vi "log analysis_gps.vi"() -> ()   [LabVIEW 2019] (continued)
INS_RTKFIXED,37.37053109061,126.72444506207,11.0879,22.3000,0.1993,-0.2262,-0.0239,-0.578200163,-2.123585690,301.384652379,0.4420,0.2933,0.5470,0.1138,0.0924,0.0770,0.0993,0.1038,4.8409,0f000001,0*2eda5995\n\t", "INSPVAXA,USB3,0,45.5,FINESTEERING,2107,282664.900,02000000,471d,15824;INS_ALIGNMENT_COMPLETE,INS_RTKFIXED,37.37053183209,126.72444381821,11.0830,22.3000,0.2025,-0.2395,-0.0183,-0.627563942,-2.176125382,301.462972604,0.4420,0.2933,0.5470,0.1138,0.0924,0.0770,0.0993,0.1038,4.8409,0f000001,0*51325076\n\t", "INSPVAXA,USB3,0,50.5,FINESTEERING,2107,282665.400,02000000,471d,15824;INS_ALIGNMENT_COMPLETE,INS_RTKFIXED,37.37053260836,126.72444247630,11.0777,22.3000,0.1697,-0.2000,-0.0233,-0.806380731,-2.428315608,301.586666898,0.4420,0.2935,0.5472,0.1137,0.0923,0.0770,0.0992,0.1038,4.8415,0f000001,0*d8a31360\n\t", "INSPVAXA,USB3,0,50.5,FINESTEERING,2107,282665.900,02000000,471d,15824;INS_ALIGNMENT_COMPLETE,INS_RTKFIXED,37.37053337130,126.72444116871,11.0726,22.3000,0.1954,-0.2209,-0.0080,-0.903161753,-2.476998563,301.699215129,0.4420,0.2935,0.5472,0.1137,0.0923,0.0770,0.0992,0.1038,4.8415,0f000001,0*b607e80f\n\t", "DUALANTENNAHEADINGA,USB3,0,47.0,FINESTEERING,2107,282666.400,02000000,d426,15824;INSUFFICIENT_OBS,NONE,-1.000000000,0.000000000,0.000000000,0.0,0.000000000,0.000000000,\"631T\",14,3,3,3,04,00,20,00*a6710081\n\t", "INSPVAXA,USB3,0,47.0,FINESTEERING,2107,282666.900,02000000,471d,15824;INS_ALIGNMENT_COMPLETE,INS_RTKFIXED,37.37053484048,126.72443859916,11.0582,22.3000,0.1830,-0.2119,-0.0311,-0.968807751,-2.464707022,301.855553753,0.4415,0.2935,0.5473,0.1137,0.0925,0.0771,0.0992,0.1038,4.8423,0f000001,0*59f4e239\n\t", "DUALANTENNAHEADINGA,USB3,0,49.5,FINESTEERING,2107,282667.400,02000000,d426,15824;INSUFFICIENT_OBS,NONE,-1.000000000,0.000000000,0.000000000,0.0,0.000000000,0.000000000,\"631T\",15,3,3,3,04,00,20,00*5f1e2af7\n\t", "INSPVAXA,USB3,0,49.5,FINESTEERING,2107,282667.900,02000000,471d,15824;INS_ALIGNMENT_COMPLETE,INS_RTKFIXED,37.37053633502,126.72443604770,11.0435,22.3000,0.1822,-0.2080,-0.0221,-0.962443537,-2.273211285,302.003209651,0.4405,0.2936,0.5472,0.1136,0.0924,0.0770,0.0991,0.1038,4.8429,0f000001,0*2d8cca71\n\t", "DUALANTENNAHEADINGA,USB3,0,51.0,FINESTEERING,2107,282668.400,02000000,d426,15824;INSUFFICIENT_OBS,NONE,-1.000000000,0.000000000,0.000000000,0.0,0.000000000,0.000000000,\"631T\",13,3,3,3,04,00,20,00*d0f86fa9\n\t", "INSPVAXA,USB3,0,51.0,FINESTEERING,2107,282668.900,02000000,471d,15824;INS_ALIGNMENT_COMPLETE,INS_RTKFIXED,37.37053784422,126.72443343900,11.0314,22.3000,0.1770,-0.2175,-0.0238,-1.067658542,-2.117354473,302.168245726,0.4406,0.2938,0.5474,0.1136,0.0926,0.0771,0.0991,0.1038,4.8433,0f000001,0*743eb533\n\t", "INSPVAXA,USB3,0,50.5,FINESTEERING,2107,282669.400,02000000,471d,15824;INS_ALIGNMENT_COMPLETE,INS_RTKFIXED,37.37053859261,126.72443216227,11.0246,22.3000,0.1748,-0.2150,-0.0262,-1.134800808,-1.987218323,302.206484559,0.4410,0.2939,0.5476,0.1137,0.0929,0.0771,0.0990,0.1039,4.8430,0f000001,0*0ef77350\n\t", "INSPVAXA,USB3,0,50.5,FINESTEERING,2107,282669.900,02000000,471d,15824;INS_ALIGNMENT_COMPLETE,INS_RTKFIXED,37.37053936070,126.72443086861,11.0170,22.3000,0.1679,-0.2152,-0.0201,-1.047863329,-2.047137616,302.259088217,0.4410,0.2939,0.5476,0.1137,0.0929,0.0771,0.0990,0.1039,4.8430,0f000001,0*b3a345e1\n\t", "INSPVAXA,USB3,0,51.5,FINESTEERING,2107,282670.400,02000000,471d,15824;INS_ALIGNMENT_COMPLETE,INS_RTKFIXED,37.37054013304,126.72442955163,11.0107,22.3000,0.1797,-0.2154,-0.0330,-1.008775367,-2.075430336,302.292083469,0.4412,0.2940,0.5477,0.1137,0.0927,0.0771,0.0989,0.1039,4.8414,0f000001,0*6124701b\n\t", "INSPVAXA,USB3,0,51.5,FINESTEERING,2107,282670.900,02000000,471d,15824;INS_ALIGNMENT_COMPLETE,INS_RTKFIXED,37.37054088934,126.72442826376,11.0051,22.3000,0.1741,-0.2301,-0.0351,-1.043464274,-1.977986056,302.323016199,0.4412,0.2940,0.5477,0.1137,0.0927,0.0771,0.0989,0.1039,4.8414,0f000001,0*5cd64784\n\t", "INSPVAXA,USB3,0,51.0,FINESTEERING,2107,282671.400,02000000,471d,15824;INS_ALIGNMENT_COMPLETE,INS_RTKFIXED,37.37054164500,126.72442698236,10.9999,22.3000,0.1651,-0.2207,-0.0264,-1.152870335,-2.003288963,302.368323626,0.4421,0.2942,0.5481,0.1138,0.0926,0.0771,0.0989,0.1039,4.8395,0f000001,0*729e65cc\n\t", "DUALANTENNAHEADINGA,USB3,0,51.0,FINESTEERING,2107,282671.900,02000000,d426,15824;SOL_COMPUTED,L1_FLOAT,-1.000000000,6.424537182,-37.266357422,0.0,360.000000000,180.000000000,\"631T\",14,5,5,5,04,00,20,20*1315aa76\n\t", "INSPVAXA,USB3,0,52.5,FINESTEERING,2107,282672.400,02000000,471d,15824;INS_ALIGNMENT_COMPLETE,INS_RTKFIXED,37.37054317479,126.72442436870,10.9904,22.3000,0.1725,-0.2321,-0.0318,-1.253314249,-1.912910767,302.408086274,0.4431,0.2945,0.5488,0.1140,0.0927,0.0771,0.0988,0.1039,4.8375,0f000001,0*4ca87b98\n\t", "INSPVAXA,USB3,0,52.5,FINESTEERING,2107,282672.900,02000000,471d,15824;INS_ALIGNMENT_COMPLETE,INS_RTKFIXED,37.37054392116,126.72442309351,10.9862,22.3000,0.1660,-0.2327,-0.0240,-1.192361701,-1.928177514,302.476152160,0.4431,0.2945,0.5488,0.1140,0.0927,0.0771,0.0988,0.1039,4.8375,0f000001,0*83cc3094\n\t", "INSPVAXA,USB3,0,51.5,FINESTEERING,2107,282673.400,02000000,471d,15824;INS_ALIGNMENT_COMPLETE,INS_RTKFIXED,37.37054468191,126.72442179361,10.9818,22.3000,0.1549,-0.2194,-0.0237,-1.138544711,-1.857754611,302.526216112,0.4445,0.2949,0.5496,0.1141,0.0925,0.0772,0.0988,0.1040,4.8352,0f000001,0*601d5af9\n\t", "INSPVAXA,USB3,0,51.5,FINESTEERING,2107,282673.900,02000000,471d,15824;INS_ALIGNMENT_COMPLETE,INS_RTKFIXED,37.37054544133,126.72442048455,10.9776,22.3000,0.1608,-0.2204,-0.0208,-1.194325383,-1.773338448,302.575514269,0.4445,0.2949,0.5496,0.1141,0.0925,0.0772,0.0988,0.1040,4.8352,0f000001,0*3c4b28bd\n\t", "DUALANTENNAHEADINGA,USB3,0,52.0,FINESTEERING,2107,282674.400,02000000,d426,15824;INSUFFICIENT_OBS,NONE,-1.000000000,0.000000000,0.000000000,0.0,0.000000000,0.000000000,\"631T\",11,3,3,3,04,00,20,00*43d09faf\n\t", "INSPVAXA,USB3,0,52.0,FINESTEERING,2107,282674.900,02000000,471d,15824;INS_ALIGNMENT_COMPLETE,INS_RTKFIXED,37.37054694617,126.72441789266,10.9675,22.3000,0.1711,-0.2297,-0.0188,-1.275138168,-1.781517765,302.710392132,0.4449,0.2948,0.5501,0.1143,0.0927,0.0772,0.0987,0.1040,4.8338,0f000001,0*704fcea3\n\t", "INSPVAXA,USB3,0,50.5,FINESTEERING,2107,282675.400,02000000,471d,15824;INS_ALIGNMENT_COMPLETE,INS_RTKFIXED,37.37054775333,126.72441659154,10.9642,22.3000,0.1645,-0.2327,-0.0094,-1.051395479,-1.879417233,302.757545593,0.4453,0.2948,0.5504,0.1142,0.0925,0.0772,0.0987,0.1040,4.8321,0f000001,0*a4c6f5d9\n\t", "DUALANTENNAHEADINGA,USB3,0,50.5,FINESTEERING,2107,282675.900,02000000,d426,15824;INSUFFICIENT_OBS,NONE,-1.000000000,0.000000000,0.000000000,0.0,0.000000000,0.000000000,\"631T\",14,3,3,3,04,00,20,00*348e632d\n\t", "INSPVAXA,USB3,0,48.5,FINESTEERING,2107,282676.400,02000000,471d,15824;INS_ALIGNMENT_COMPLETE,INS_RTKFIXED,37.37054934080,126.72441402594,10.9604,22.3000,0.1664,-0.2342,-0.0147,-1.030303751,-1.986468861,302.910679697,0.4460,0.2946,0.5508,0.1143,0.0923,0.0772,0.0987,0.1040,4.8310,0f000001,0*713be666\n\t", "INSPVAXA,USB3,0,48.5,FINESTEERING,2107,282676.900,02000000,471d,15824;INS_ALIGNMENT_COMPLETE,INS_RTKFIXED,37.37055013334,126.72441273552,10.9584,22.3000,0.1604,-0.2244,-0.0102,-1.040479369,-1.905860693,302.964821011,0.4460,0.2946,0.5508,0.1143,0.0923,0.0772,0.0987,0.1040,4.8310,0f000001,0*b8bc8b15\n\t", "INSPVAXA,USB3,0,50.5,FINESTEERING,2107,282677.400,02000000,471d,15824;INS_ALIGNMENT_COMPLETE,INS_RTKFIXED,37.37055094880,126.72441141455,10.9545,22.3000,0.1625,-0.2172,-0.0160,-0.890769170,-1.829812831,303.004445292,0.4467,0.2944,0.5513,0.1144,0.0924,0.0772,0.0987,0.1040,4.8309,0f000001,0*53662f9b\n\t", "DUALANTENNAHEADINGA,USB3,0,50.5,FINESTEERING,2107,282677.900,02000000,d426,15824;INSUFFICIENT_OBS,NONE,-1.000000000,0.000000000,0.000000000,0.0,0.000000000,0.000000000,\"631T\",15,3,3,3,04,00,20,00*38dceac7\n\t", "INSPVAXA,USB3,0,43.0,FINESTEERING,2107,282678.400,02000000,471d,15824;INS_ALIGNMENT_COMPLETE,INS_RTKFIXED,37.37055255572,126.72440886198,10.9468,22.3000,0.1687,-0.2243,-0.0108,-0.678924233,-1.833067267,303.044860891,0.4469,0.2942,0.5516,0.1145,0.0924,0.0772,0.0987,0.1040,4.8313,0f000001,0*bb99175a\n\t", "DUALANTENNAHEADINGA,USB3,0,43.0,FINESTEERING,2107,282678.900,02000000,d426,15824;INSUFFICIENT_OBS,NONE,-1.000000000,0.000000000,0.000000000,0.0,0.000000000,0.000000000,\"631T\",14,3,3,3,04,00,20,00*c50de69c\n\t", "DUALANTENNAHEADINGA,USB3,0,51.0,FINESTEERING,2107,282679.400,02000000,d426,15824;SOL_COMPUTED,L1_FLOAT,-1.000000000,21.335779190,-47.169494629,0.0,193.181869507,129.996200562,\"631T\",14,5,5,5,04,00,20,20*2871a391\n\t", "DUALANTENNAHEADINGA,USB3,0,51.0,FINESTEERING,2107,282679.900,02000000,d426,15824;SOL_COMPUTED,L1_FLOAT,-1.000000000,20.963815689,-49.860382080,0.0,193.921173096,108.310935974,\"631T\",14,5,5,5,04,00,20,20*13dab214\n\t", "INSPVAXA,USB3,0,49.5,FINESTEERING,2107,282680.400,02000000,471d,15824;INS_ALIGNMENT_COMPLETE,INS_RTKFIXED,37.37055584590,126.72440372212,10.9267,22.3000,0.1683,-0.2234,-0.0175,-0.724680252,-2.288934243,303.019606078,0.4465,0.2938,0.5517,0.1142,0.0925,0.0772,0.0987,0.1039,4.8325,0f000001,0*ef175975\n\t", "DUALANTENNAHEADINGA,USB3,0,49.5,FINESTEERING,2107,282680.900,02000000,d426,15824;SOL_COMPUTED,L1_FLOAT,-1.000000000,17.254264832,-46.720001221,0.0,249.251464844,160.460342407,\"631T\",15,5,5,5,04,00,20,20*4935c559\n\t", "DUALANTENNAHEADINGA,USB3,0,52.0,FINESTEERING,2107,282681.400,02000000,d426,15824;SOL_COMPUTED,L1_FLOAT,-1.000000000,5.197163105,-35.837677002,0.0,360.000000000,180.000000000,\"631T\",15,5,5,5,04,00,20,20*e552e6d0\n\t", "DUALANTENNAHEADINGA,USB3,0,52.0,FINESTEERING,2107,282681.900,02000000,d426,15824;SOL_COMPUTED,L1_FLOAT,-1.000000000,5.226606846,-33.722320557,0.0,360.000000000,180.000000000,\"631T\",14,5,5,5,04,00,20,20*81528f45\n\t", "DUALANTENNAHEADINGA,USB3,0,46.5,FINESTEERING,2107,282682.400,02000000,d426,15824;SOL_COMPUTED,L1_FLOAT,-1.000000000,356.926879883,-21.442382813,0.0,360.000000000,180.000000000,\"631T\",14,5,5,5,04,00,20,20*df144227\n\t", "DUALANTENNAHEADINGA,USB3,0,46.5,FINESTEERING,2107,282682.900,02000000,d426,15824;SOL_COMPUTED,L1_FLOAT,-1.000000000,355.913299561,-34.093353271,0.0,360.000000000,180.000000000,\"631T\",16,5,5,5,04,00,20,20*8a484d88\n\t", "INSPVAXA,USB3,0,47.5,FINESTEERING,2107,282683.400,02008000,471d,15824;INS_ALIGNMENT_COMPLETE,INS_RTKFIXED,37.37056070988,126.72439621643,10.8934,22.3000,0.1823,-0.2154,-0.0338,-0.633682870,-1.700441469,302.701865848,0.4459,0.2937,0.5514,0.1144,0.0924,0.0772,0.0987,0.1039,4.8335,0f000001,0*fab402d9\n\t", "INSPVAXA,USB3,0,47.5,FINESTEERING,2107,282683.900,02008000,471d,15824;INS_ALIGNMENT_COMPLETE,INS_RTKFIXED,37.37056151412,126.72439497192,10.8876,22.3000,0.1856,-0.2259,-0.0357,-0.593256165,-1.575198052,302.563875130,0.4459,0.2937,0.5514,0.1144,0.0924,0.0772,0.0987,0.1039,4.8335,0f000001,0*6eaca9c0\n\t", "DUALANTENNAHEADINGA,USB3,0,48.0,FINESTEERING,2107,282684.400,02008000,d426,15824;INSUFFICIENT_OBS,NONE,-1.000000000,0.000000000,0.000000000,0.0,0.000000000,0.000000000,\"631T\",14,3,3,3,04,00,20,00*e1343e52\n\t", "DUALANTENNAHEADINGA,USB3,0,48.0,FINESTEERING,2107,282684.900,02008000,d426,15824;INSUFFICIENT_OBS,NONE,-1.000000000,0.000000000,0.000000000,0.0,0.000000000,0.000000000,\"631T\",14,3,3,3,04,00,20,00*58cb0037\n\t", "DUALANTENNAHEADINGA,USB3,0,50.0,FINESTEERING,2107,282685.400,02008000,d426,15824;INSUFFICIENT_OBS,NONE,-1.000000000,0.000000000,0.000000000,0.0,0.000000000,0.000000000,\"631T\",15,3,3,3,04,00,20,00*1e152056\n\t", "DUALANTENNAHEADINGA,USB3,0,50.0,FINESTEERING,2107,282685.900,02008000,d426,15824;INSUFFICIENT_OBS,NONE,-1.000000000,0.000000000,0.000000000,0.0,0.000000000,0.000000000,\"631T\",15,3,3,3,04,00,20,00*a7ea1e33\n\t", "INSPVAXA,USB3,0,47.0,FINESTEERING,2107,282686.400,02008000,471d,15824;INS_ALIGNMENT_COMPLETE,INS_RTKFIXED,37.37056557594,126.72438871297,10.8671,22.3000,0.1902,-0.2071,-0.0220,-0.466180041,-1.620819685,301.862974006,0.4463,0.2937,0.5510,0.1145,0.0924,0.0772,0.0987,0.1039,4.8334,0f000001,0*000637b1\n\t", "DUALANTENNAHEADINGA,USB3,0,47.0,FINESTEERING,2107,282686.900,02008000,d426,15824;INSUFFICIENT_OBS,NONE,-1.000000000,0.000000000,0.000000000,0.0,0.000000000,0.000000000,\"631T\",15,3,3,3,04,00,20,00*26f21742\n\t", "DUALANTENNAHEADINGA,USB3,0,48.0,FINESTEERING,2107,282687.400,02000000,d426,15824;INSUFFICIENT_OBS,NONE,-1.000000000,0.000000000,0.000000000,0.0,0.000000000,0.000000000,\"631T\",15,3,3,3,04,00,20,00*962d37c0\n\t", "INSPVAXA,USB3,0,48.0,FINESTEERING,2107,282687.900,02000000,471d,15824;INS_ALIGNMENT_COMPLETE,INS_RTKFIXED,37.37056796292,126.72438494002,10.8533,22.3000,0.1859,-0.2072,-0.0348,-0.193858234,-1.879869364,301.375328735,0.4457,0.2937,0.5507,0.1142,0.0925,0.0771,0.0987,0.1038,4.8329,0f000001,0*d3beefd5\n\t", "DUALANTENNAHEADINGA,USB3,0,47.0,FINESTEERING,2107,282688.400,02000000,d426,15824;INSUFFICIENT_OBS,NONE,-1.000000000,0.000000000,0.000000000,0.0,0.000000000,0.000000000,\"631T\",13,3,3,3,04,00,20,00*7bc19048\n\t", "DUALANTENNAHEADINGA,USB3,0,47.0,FINESTEERING,2107,282688.900,02000000,d426,15824;INSUFFICIENT_OBS,NONE,-1.000000000,0.000000000,0.000000000,0.0,0.000000000,0.000000000,\"631T\",16,3,3,3,04,00,20,00*fcb42397\n\t", "DUALANTENNAHEADINGA,USB3,0,48.0,FINESTEERING,2107,282689.400,02000000,d426,15824;INSUFFICIENT_OBS,NONE,-1.000000000,0.000000000,0.000000000,0.0,0.000000000,0.000000000,\"631T\",16,3,3,3,04,00,20,00*5af887b4\n\t", "DUALANTENNAHEADINGA,USB3,0,48.0,FINESTEERING,2107,282689.900,02000000,d426,15824;INSUFFICIENT_OBS,NONE,-1.000000000,0.000000000,0.000000000,0.0,0.000000000,0.000000000,\"631T\",14,3,3,3,04,00,20,00*97b3bf20\n\t", "DUALANTENNAHEADINGA,USB3,0,52.0,FINESTEERING,2107,282690.400,02000000,d426,15824;INSUFFICIENT_OBS,NONE,-1.000000000,0.000000000,0.000000000,0.0,0.000000000,0.000000000,\"631T\",13,3,3,3,04,00,20,00*a378a124\n\t", "DUALANTENNAHEADINGA,USB3,0,52.0,FINESTEERING,2107,282690.900,02000000,d426,15824;INSUFFICIENT_OBS,NONE,-1.000000000,0.000000000,0.000000000,0.0,0.000000000,0.000000000,\"631T\",14,3,3,3,04,00,20,00*50b9140a\n\t", "DUALANTENNAHEADINGA,USB3,0,51.5,FINESTEERING,2107,282691.400,02000000,d426,15824;INSUFFICIENT_OBS,NONE,-1.000000000,0.000000000,0.000000000,0.0,0.000000000,0.000000000,\"631T\",16,3,3,3,04,00,20,00*099db567\n\t", "DUALANTENNAHEADINGA,USB3,0,51.5,FINESTEERING,2107,282691.900,02000000,d426,15824;INSUFFICIENT_OBS,NONE,-1.000000000,0.000000000,0.000000000,0.0,0.000000000,0.000000000,\"631T\",16,3,3,3,04,00,20,00*b0628b02\n\t", "DUALANTENNAHEADINGA,USB3,0,50.5,FINESTEERING,2107,282692.400,02000000,d426,15824;INSUFFICIENT_OBS,NONE,-1.000000000,0.000000000,0.000000000,0.0,0.000000000,0.000000000,\"631T\",16,3,3,3,04,00,20,00*dbb16ea8\n\t", "DUALANTENNAHEADINGA,USB3,0,50.5,FINESTEERING,2107,282692.900,02000000,d426,15824;INSUFFICIENT_OBS,NONE,-1.000000000,0.000000000,0.000000000,0.0,0.000000000,0.000000000,\"631T\",16,3,3,3,04,00,20,00*624e50cd\n\t", "DUALANTENNAHEADINGA,USB3,0,49.5,FINESTEERING,2107,282693.400,02000000,d426,15824;INSUFFICIENT_OBS,NONE,-1.000000000,0.000000000,0.000000000,0.0,0.000000000,0.000000000,\"631T\",16,3,3,3,04,00,20,00*97362650\n\t", "DUALANTENNAHEADINGA,USB3,0,49.5,FINESTEERING,2107,282694.400,02000000,d426,15824;INSUFFICIENT_OBS,NONE,-1.000000000,0.000000000,0.000000000,0.0,0.000000000,0.000000000,\"631T\",16,3,3,3,04,00,20,00*4d4f3e1e\n\t", "DUALANTENNAHEADINGA,USB3,0,49.5,FINESTEERING,2107,282694.900,02000000,d426,15824;INSUFFICIENT_OBS,NONE,-1.000000000,0.000000000,0.000000000,0.0,0.000000000,0.000000000,\"631T\",16,3,3,3,04,00,20,00*f4b0007b\n\t", "DUALANTENNAHEADINGA,USB3,0,47.5,FINESTEERING,2107,282695.400,02000000,d426,15824;INSUFFICIENT_OBS,NONE,-1.000000000,0.000000000,0.000000000,0.0,0.000000000,0.000000000,\"631T\",15,3,3,3,04,00,20,00*95eef455\n\t", "DUALANTENNAHEADINGA,USB3,0,47.5,FINESTEERING,2107,282695.900,02000000,d426,15824;INSUFFICIENT_OBS,NONE,-1.000000000,0.000000000,0.000000000,0.0,0.000000000,0.000000000,\"631T\",15,3,3,3,04,00,20,00*2c11ca30\n\t", "DUALANTENNAHEADINGA,USB3,0,48.0,FINESTEERING,2107,282696.400,02000000,d426,15824;INSUFFICIENT_OBS,NONE,-1.000000000,0.000000000,0.000000000,0.0,0.000000000,0.000000000,\"631T\",15,3,3,3,04,00,20,00*0497816d\n\t", "DUALANTENNAHEADINGA,USB3,0,48.0,FINESTEERING,2107,282696.900,02000000,d426,15824;INSUFFICIENT_OBS,NONE,-1.000000000,0.000000000,0.000000000,0.0,0.000000000,0.000000000,\"631T\",16,3,3,3,04,00,20,00*1e3e39a1\n\t", "DUALANTENNAHEADINGA,USB3,0,47.0,FINESTEERING,2107,282697.900,02000000,d426,15824;INSUFFICIENT_OBS,NONE,-1.000000000,0.000000000,0.000000000,0.0,0.000000000,0.000000000,\"631T\",18,3,3,3,04,00,20,00*95f0b571\n\t", "DUALANTENNAHEADINGA,USB3,0,50.0,FINESTEERING,2107,282698.400,02000000,d426,15824;INSUFFICIENT_OBS,NONE,-1.000000000,0.000000000,0.000000000,0.0,0.000000000,0.000000000,\"631T\",17,3,3,3,04,00,20,00*5abb2bc4\n\t", "DUALANTENNAHEADINGA,USB3,0,50.0,FINESTEERING,2107,282698.900,02000000,d426,15824;INSUFFICIENT_OBS,NONE,-1.000000000,0.000000000,0.000000000,0.0,0.000000000,0.000000000,\"631T\",17,3,3,3,04,00,20,00*e34415a1\n\t", "DUALANTENNAHEADINGA,USB3,0,52.0,FINESTEERING,2107,282699.400,02000000,d426,15824;INSUFFICIENT_OBS,NONE,-1.000000000,0.000000000,0.000000000,0.0,0.000000000,0.000000000,\"631T\",17,3,3,3,04,00,20,00*ffea8255\n\t", "DUALANTENNAHEADINGA,USB3,0,52.0,FINESTEERING,2107,282699.900,02000000,d426,15824;INSUFFICIENT_OBS,NONE,-1.000000000,0.000000000,0.000000000,0.0,0.000000000,0.000000000,\"631T\",17,3,3,3,04,00,20,00*4615bc30\n\t", "DUALANTENNAHEADINGA,USB3,0,50.0,FINESTEERING,2107,282700.400,02000000,d426,15824;INSUFFICIENT_OBS,NONE,-1.000000000,0.000000000,0.000000000,0.0,0.000000000,0.000000000,\"631T\",12,3,3,3,04,00,20,00*82376373\n\t", "DUALANTENNAHEADINGA,USB3,0,50.0,FINESTEERING,2107,282700.900,02000000,d426,15824;INSUFFICIENT_OBS,NONE,-1.000000000,0.000000000,0.000000000,0.0,0.000000000,0.000000000,\"631T\",12,3,3,3,04,00,20,00*3bc85d16\n\t", "INSPVAXA,USB3,0,51.0,FINESTEERING,2107,282701.950,02000000,471d,15824;INS_ALIGNMENT_COMPLETE,INS_RTKFIXED,37.37058966654,126.72434893958,10.7130,22.3000,0.1917,-0.1995,-0.0321,0.078081092,-1.836601738,301.669382711,0.4402,0.2934,0.5473,0.1136,0.0923,0.0770,0.0988,0.1035,4.8261,0f000001,0*8e2fcc51\n\t", "DUALANTENNAHEADINGA,USB3,0,51.0,FINESTEERING,2107,282702.900,02000000,d426,15824;INSUFFICIENT_OBS,NONE,-1.000000000,0.000000000,0.000000000,0.0,0.000000000,0.000000000,\"631T\",15,3,3,3,04,00,20,00*ce02094b\n\t", "INSPVAXA,USB3,0,51.0,FINESTEERING,2107,282703.450,02000000,471d,15824;INS_ALIGNMENT_COMPLETE,INS_RTKFIXED,37.37059201506,126.72434506763,10.7048,22.3000,0.1803,-0.1856,-0.0247,-0.105787498,-1.952133227,301.410927421,0.4394,0.2932,0.5469,0.1134,0.0923,0.0770,0.0988,0.1035,4.8271,0f000001,0*f23aaa81\n\t", "INSPVAXA,USB3,0,51.0,FINESTEERING,2107,282703.950,02000000,471d,15824;INS_ALIGNMENT_COMPLETE,INS_RTKFIXED,37.37059277883,126.72434379347,10.7003,22.3000,0.1861,-0.1882,-0.0190,-0.127062602,-1.998823020,301.296665228,0.4394,0.2932,0.5469,0.1134,0.0923,0.0770,0.0988,0.1035,4.8271,0f000001,0*9cb21e47\n\t", "INSPVAXA,USB3,0,45.5,FINESTEERING,2107,282704.450,02000000,471d,15824;INS_ALIGNMENT_COMPLETE,INS_RTKFIXED,37.37059354994,126.72434248772,10.6964,22.3000,0.1805,-0.1784,-0.0168,-0.125494848,-2.044475931,301.198188226,0.4393,0.2932,0.5468,0.1133,0.0923,0.0770,0.0987,0.1035,4.8275,0f000001,0*dae1e343\n\t", "INSPVAXA,USB3,0,45.5,FINESTEERING,2107,282704.950,02000000,471d,15824;INS_ALIGNMENT_COMPLETE,INS_RTKFIXED,37.37059432216,126.72434118765,10.6925,22.3000,0.1836,-0.2007,-0.0268,-0.089569807,-2.221768291,301.087967534,0.4393,0.2932,0.5468,0.1133,0.0923,0.0770,0.0987,0.1035,4.8275,0f000001,0*2b6d582c\n\t", "DUALANTENNAHEADINGA,USB3,0,48.5,FINESTEERING,2107,282705.400,02000000,d426,15824;INSUFFICIENT_OBS,NONE,-1.000000000,0.000000000,0.000000000,0.0,0.000000000,0.000000000,\"631T\",14,3,3,3,04,00,20,00*0e4305d5\n\t", "DUALANTENNAHEADINGA,USB3,0,48.5,FINESTEERING,2107,282705.900,02000000,d426,15824;INSUFFICIENT_OBS,NONE,-1.000000000,0.000000000,0.000000000,0.0,0.000000000,0.000000000,\"631T\",14,3,3,3,04,00,20,00*b7bc3bb0\n\t", "INSPVAXA,USB3,0,47.5,FINESTEERING,2107,282706.450,02000000,471d,15824;INS_ALIGNMENT_COMPLETE,INS_RTKFIXED,37.37059659513,126.72433727332,10.6837,22.3000,0.1676,-0.1882,-0.0314,-0.220175283,-2.295370003,300.572862367,0.4389,0.2931,0.5466,0.1133,0.0923,0.0770,0.0987,0.1035,4.8288,0f000001,0*8941e111\n\t", "DUALANTENNAHEADINGA,USB3,0,47.5,FINESTEERING,2107,282706.900,02000000,d426,15824;INSUFFICIENT_OBS,NONE,-1.000000000,0.000000000,0.000000000,0.0,0.000000000,0.000000000,\"631T\",11,3,3,3,04,00,20,00*4d3525fe\n\t", "DUALANTENNAHEADINGA,USB3,0,52.0,FINESTEERING,2107,282707.400,02000000,d426,15824;INSUFFICIENT_OBS,NONE,-1.000000000,0.000000000,0.000000000,0.0,0.000000000,0.000000000,\"631T\",12,3,3,3,04,00,20,00*90c7d675\n\t", "DUALANTENNAHEADINGA,USB3,0,52.0,FINESTEERING,2107,282707.900,02000000,d426,15824;INSUFFICIENT_OBS,NONE,-1.000000000,0.000000000,0.000000000,0.0,0.000000000,0.000000000,\"631T\",13,3,3,3,04,00,20,00*feda6848\n\t", "DUALANTENNAHEADINGA,USB3,0,52.0,FINESTEERING,2107,282708.900,02000000,d426,15824;INSUFFICIENT_OBS,NONE,-1.000000000,0.000000000,0.000000000,0.0,0.000000000,0.000000000,\"631T\",15,3,3,3,04,00,20,00*615d515f\n\t", "INSPVAXA,USB3,0,46.5,FINESTEERING,2107,282709.450,02000000,471d,15824;INS_ALIGNMENT_COMPLETE,INS_RTKFIXED,37.37060113294,126.72432942720,10.6558,22.3000,0.1792,-0.2126,-0.0198,-0.200491468,-1.971404566,300.268575337,0.4402,0.2931,0.5474,0.1135,0.0922,0.0770,0.0986,0.1035,4.8320,0f000001,0*91b882c4\n\t", "DUALANTENNAHEADINGA,USB3,0,46.5,FINESTEERING,2107,282709.900,02000000,d426,15824;INSUFFICIENT_OBS,NONE,-1.000000000,0.000000000,0.000000000,0.0,0.000000000,0.000000000,\"631T\",13,3,3,3,04,00,20,00*5f9ec7af\n\t", "INSPVAXA,USB3,0,46.5,FINESTEERING,2107,282710.450,02000000,471d,15824;INS_ALIGNMENT_COMPLETE,INS_RTKFIXED,37.37060265280,126.72432675986,10.6463,22.3000,0.1745,-0.2044,-0.0168,-0.207189444,-2.098625918,300.356289546,0.4398,0.2931,0.5473,0.1134,0.0922,0.0770,0.0986,0.1035,4.8333,0f000001,0*cf6a9f79\n\t", "INSPVAXA,USB3,0,47.5,FINESTEERING,2107,282711.450,02000000,471d,15824;INS_ALIGNMENT_COMPLETE,INS_RTKFIXED,37.37060415509,126.72432413204,10.6400,22.3000,0.1796,-0.1977,-0.0235,-0.256481556,-2.212753880,300.512449739,0.4392,0.2930,0.5470,0.1133,0.0922,0.0770,0.0986,0.1035,4.8345,0f000001,0*c0ba1218\n\t", "INSPVAXA,USB3,0,47.5,FINESTEERING,2107,282712.450,02000000,471d,15824;INS_ALIGNMENT_COMPLETE,INS_RTKFIXED,37.37060568585,126.72432146015,10.6310,22.3000,0.1690,-0.1966,-0.0239,-0.257627218,-1.930020339,300.742925306,0.4385,0.2930,0.5468,0.1132,0.0922,0.0770,0.0986,0.1035,4.8358,0f000001,0*254ba6dd\n\t", "INSPVAXA,USB3,0,48.0,FINESTEERING,2107,282713.450,02000000,471d,15824;INS_ALIGNMENT_COMPLETE,INS_RTKFIXED,37.37060718735,126.72431885308,10.6223,22.3000,0.1755,-0.2010,-0.0238,-0.293375076,-1.794770522,300.954779767,0.4381,0.2930,0.5465,0.1133,0.0923,0.0770,0.0986,0.1035,4.8370,0f000001,0*2485d43a\n\t", "DUALANTENNAHEADINGA,USB3,0,48.0,FINESTEERING,2107,282713.900,02000000,d426,15824;INSUFFICIENT_OBS,NONE,-1.000000000,0.000000000,0.000000000,0.0,0.000000000,0.000000000,\"631T\",15,3,3,3,04,00,20,00*7de7f3c7\n\t", "INSPVAXA,USB3,0,50.5,FINESTEERING,2107,282714.450,02000000,471d,15824;INS_ALIGNMENT_COMPLETE,INS_RTKFIXED,37.37060872505,126.72431621182,10.6168,22.3000,0.1744,-0.1980,-0.0186,-0.254099040,-1.809317915,301.200596990,0.4382,0.2930,0.5463,0.1133,0.0922,0.0770,0.0986,0.1035,4.8379,0f000001,0*a4919b29\n\t", "INSPVAXA,USB3,0,50.5,FINESTEERING,2107,282714.950,02000000,471d,15824;INS_ALIGNMENT_COMPLETE,INS_RTKFIXED,37.37060951512,126.72431487294,10.6136,22.3000,0.1802,-0.2114,-0.0189,-0.186867307,-1.902236696,301.349579343,0.4382,0.2930,0.5463,0.1133,0.0922,0.0770,0.0986,0.1035,4.8379,0f000001,0*eb262157\n\t", "INSPVAXA,USB3,0,51.5,FINESTEERING,2107,282715.450,02000000,471d,15824;INS_ALIGNMENT_COMPLETE,INS_RTKFIXED,37.37061032466,126.72431346163,10.6103,22.3000,0.1848,-0.2311,-0.0198,-0.404081193,-1.989525185,301.491166671,0.4382,0.2930,0.5462,0.1132,0.0922,0.0770,0.0986,0.1035,4.8387,0f000001,0*760e8d75\n\t", "INSPVAXA,USB3,0,45.5,FINESTEERING,2107,282716.450,02000000,471d,15824;INS_ALIGNMENT_COMPLETE,INS_RTKFIXED,37.37061184609,126.72431094127,10.6047,22.3000,0.1655,-0.1918,-0.0154,-0.319182162,-2.031673145,301.719710167,0.4383,0.2930,0.5462,0.1134,0.0922,0.0770,0.0985,0.1035,4.8397,0f000001,0*42f3853e\n\t", "DUALANTENNAHEADINGA,USB3,0,47.5,FINESTEERING,2107,282717.400,02000000,d426,15824;INSUFFICIENT_OBS,NONE,-1.000000000,0.000000000,0.000000000,0.0,0.000000000,0.000000000,\"631T\",14,3,3,3,04,00,20,00*58fa208c\n\t", "INSPVAXA,USB3,0,51.0,FINESTEERING,2107,282718.450,02000000,471d,15824;INS_ALIGNMENT_COMPLETE,INS_RTKFIXED,37.37061503275,126.72430567052,10.5915,22.3000,0.1670,-0.2003,-0.0156,-0.481720437,-1.537833901,302.225440084,0.4384,0.2930,0.5461,0.1133,0.0922,0.0770,0.0985,0.1035,4.8414,0f000001,0*c2621da1\n\t", "INSPVAXA,USB3,0,50.5,FINESTEERING,2107,282719.450,02000000,471d,15824;INS_ALIGNMENT_COMPLETE,INS_RTKFIXED,37.37061661000,126.72430311428,10.5856,22.3000,0.1775,-0.2289,-0.0225,-0.409943136,-1.702424996,302.531013260,0.4388,0.2931,0.5463,0.1134,0.0923,0.0770,0.0985,0.1035,4.8421,0f000001,0*cccf0b07\n\t", "INSPVAXA,USB3,0,50.5,FINESTEERING,2107,282719.950,02000000,471d,15824;INS_ALIGNMENT_COMPLETE,INS_RTKFIXED,37.37061741122,126.72430179575,10.5834,22.3000,0.1586,-0.2047,-0.0162,-0.368316866,-1.792689997,302.616582659,0.4388,0.2931,0.5463,0.1134,0.0923,0.0770,0.0985,0.1035,4.8421,0f000001,0*6a624589\n\t", "INSPVAXA,USB3,0,52.5,FINESTEERING,2107,282720.450,02000000,471d,15824;INS_ALIGNMENT_COMPLETE,INS_RTKFIXED,37.37061822096,126.72430049242,10.5799,22.3000,0.1755,-0.2081,-0.0186,-0.303677811,-1.979848270,302.687255780,0.4391,0.2932,0.5464,0.1134,0.0923,0.0770,0.0985,0.1035,4.8427,0f000001,0*d8d179e3\n\t", "INSPVAXA,USB3,0,52.5,FINESTEERING,2107,282720.950,02000000,471d,15824;INS_ALIGNMENT_COMPLETE,INS_RTKFIXED,37.37061900063,126.72429922706,10.5769,22.3000,0.1781,-0.2246,-0.0135,-0.518744343,-1.838149425,302.751038564,0.4391,0.2932,0.5464,0.1134,0.0923,0.0770,0.0985,0.1035,4.8427,0f000001,0*0bb3f92c\n\t", "INSPVAXA,USB3,0,50.0,FINESTEERING,2107,282721.450,02000000,471d,15824;INS_ALIGNMENT_COMPLETE,INS_RTKFIXED,37.37061979310,126.72429796144,10.5749,22.3000,0.1738,-0.2158,-0.0193,-0.356246075,-1.735257546,302.750930181,0.4391,0.2932,0.5464,0.1133,0.0922,0.0770,0.0985,0.1035,4.8432,0f000001,0*0b05b843\n\t", "INSPVAXA,USB3,0,50.0,FINESTEERING,2107,282721.950,02000000,471d,15824;INS_ALIGNMENT_COMPLETE,INS_RTKFIXED,37.37062058978,126.72429668610,10.5720,22.3000,0.1774,-0.2184,-0.0211,-0.236483678,-1.725198651,302.717948727,0.4391,0.2932,0.5464,0.1133,0.0922,0.0770,0.0985,0.1035,4.8432,0f000001,0*43a1a225\n\t", "INSPVAXA,USB3,0,52.5,FINESTEERING,2107,282722.450,02000000,471d,15824;INS_ALIGNMENT_COMPLETE,INS_RTKFIXED,37.37062139294,126.72429536987,10.5676,22.3000,0.1685,-0.2034,-0.0272,-0.122026198,-1.692741983,302.685736194,0.4390,0.2932,0.5464,0.1133,0.0922,0.0770,0.0985,0.1034,4.8438,0f000001,0*76333eb5\n\t", "INSPVAXA,USB3,0,52.5,FINESTEERING,2107,282722.950,02000000,471d,15824;INS_ALIGNMENT_COMPLETE,INS_RTKFIXED,37.37062216038,126.72429408931,10.5632,22.3000,0.1618,-0.2145,-0.0280,-0.230140529,-1.688611156,302.634243103,0.4390,0.2932,0.5464,0.1133,0.0922,0.0770,0.0985,0.1034,4.8438,0f000001,0*93bbad2f\n\t", "INSPVAXA,USB3,0,49.5,FINESTEERING,2107,282723.950,02000000,471d,15824;INS_ALIGNMENT_COMPLETE,INS_RTKFIXED,37.37062369834,126.72429151405,10.5583,22.3000,0.1641,-0.2086,-0.0359,-0.178637148,-1.711321137,302.326470730,0.4391,0.2932,0.5465,0.1133,0.0923,0.0770,0.0985,0.1034,4.8445,0f000001,0*3c6720b9\n\t", "INSPVAXA,USB3,0,45.0,FINESTEERING,2107,282724.450,02000000,471d,15824;INS_ALIGNMENT_COMPLETE,INS_RTKFIXED,37.37062445195,126.72429020244,10.5541,22.3000,0.1656,-0.2090,-0.0302,-0.201495719,-1.654592110,302.120912314,0.4391,0.2932,0.5466,0.1133,0.0923,0.0770,0.0985,0.1034,4.8452,0f000001,0*d09f31ec\n\t", "INSPVAXA,USB3,0,45.0,FINESTEERING,2107,282724.950,02000000,471d,15824;INS_ALIGNMENT_COMPLETE,INS_RTKFIXED,37.37062519689,126.72428891232,10.5496,22.3000,0.1594,-0.2061,-0.0364,-0.113683805,-1.562683134,301.999815122,0.4391,0.2932,0.5466,0.1133,0.0923,0.0770,0.0985,0.1034,4.8452,0f000001,0*065bc9da\n\t", "INSPVAXA,USB3,0,52.5,FINESTEERING,2107,282725.450,02000000,471d,15824;INS_ALIGNMENT_COMPLETE,INS_RTKFIXED,37.37062594102,126.72428759328,10.5455,22.3000,0.1686,-0.2211,-0.0237,-0.147215314,-1.711523194,301.868011628,0.4387,0.2932,0.5466,0.1133,0.0923,0.0770,0.0985,0.1034,4.8461,0f000001,0*ee4f0d81\n\t", "INSPVAXA,USB3,0,52.5,FINESTEERING,2107,282725.950,02000000,471d,15824;INS_ALIGNMENT_COMPLETE,INS_RTKFIXED,37.37062668932,126.72428627001,10.5411,22.3000,0.1745,-0.2284,-0.0369,-0.083032064,-1.696566260,301.720636014,0.4387,0.2932,0.5466,0.1133,0.0923,0.0770,0.0985,0.1034,4.8461,0f000001,0*1eb70b76\n\t", "INSPVAXA,USB3,0,51.5,FINESTEERING,2107,282726.950,02000000,471d,15824;INS_ALIGNMENT_COMPLETE,INS_RTKFIXED,37.37062817613,126.72428365004,10.5325,22.3000,0.1755,-0.2305,-0.0299,-0.122209734,-1.767911685,301.603525857,0.4391,0.2932,0.5469,0.1133,0.0923,0.0770,0.0985,0.1034,4.8469,0f000001,0*3fbc9b25\n\t", "INSPVAXA,USB3,0,51.0,FINESTEERING,2107,282727.450,02000000,471d,15824;INS_ALIGNMENT_COMPLETE,INS_RTKFIXED,37.37062893743,126.72428230772,10.5272,22.3000,0.1765,-0.2181,-0.0244,-0.186365887,-1.943545299,301.556542913,0.4394,0.2932,0.5472,0.1133,0.0923,0.0770,0.0985,0.1034,4.8480,0f000001,0*c4ce36d4\n\t", "INSPVAXA,USB3,0,51.0,FINESTEERING,2107,282727.950,02000000,471d,15824;INS_ALIGNMENT_COMPLETE,INS_RTKFIXED,37.37062969227,126.72428097983,10.5215,22.3000,0.1787,-0.2040,-0.0183,-0.254427310,-1.978392002,301.576926117,0.4394,0.2932,0.5472,0.1133,0.0923,0.0770,0.0985,0.1034,4.8480,0f000001,0*e99e732b\n\t", "INSPVAXA,USB3,0,51.5,FINESTEERING,2107,282728.950,02000000,471d,15824;INS_ALIGNMENT_COMPLETE,INS_RTKFIXED,37.37063122299,126.72427838355,10.5148,22.3000,0.1885,-0.2208,-0.0203,-0.119828900,-1.930080778,301.638982245,0.4399,0.2933,0.5477,0.1134,0.0923,0.0770,0.0984,0.1034,4.8492,0f000001,0*2b605f5c\n\t", "INSPVAXA,USB3,0,52.5,FINESTEERING,2107,282729.950,02000000,471d,15824;INS_ALIGNMENT_COMPLETE,INS_RTKFIXED,37.37063278846,126.72427577866,10.5058,22.3000,0.1873,-0.2222,-0.0212,-0.280509981,-1.724312983,301.915248261,0.4403,0.2933,0.5480,0.1134,0.0923,0.0770,0.0984,0.1035,4.8506,0f000001,0*b7f0a5a5\n\t", "INSPVAXA,USB3,0,51.5,FINESTEERING,2107,282730.450,02000000,471d,15824;INS_ALIGNMENT_COMPLETE,INS_RTKFIXED,37.37063357878,126.72427449323,10.5033,22.3000,0.1727,-0.2057,-0.0242,-0.264377135,-1.835119150,302.025936707,0.4422,0.2933,0.5491,0.1137,0.0923,0.0771,0.0985,0.1035,4.8518,0f000001,0*7f6e5cf1\n\t", "INSPVAXA,USB3,0,49.0,FINESTEERING,2107,282731.450,02000000,471d,15824;INS_ALIGNMENT_COMPLETE,INS_RTKFIXED,37.37063518922,126.72427189807,10.4972,22.3000,0.1874,-0.2156,-0.0321,-0.243858308,-2.166120506,302.258331909,0.4432,0.2934,0.5498,0.1138,0.0924,0.0771,0.0985,0.1035,4.8531,0f000001,0*8b4646cd\n\t", "INSPVAXA,USB3,0,49.0,FINESTEERING,2107,282731.950,02000000,471d,15824;INS_ALIGNMENT_COMPLETE,INS_RTKFIXED,37.37063597309,126.72427066217,10.4933,22.3000,0.1763,-0.1976,-0.0267,-0.212826377,-2.311379439,302.361551522,0.4432,0.2934,0.5498,0.1138,0.0924,0.0771,0.0985,0.1035,4.8531,0f000001,0*776c7422\n\t", "INSPVAXA,USB3,0,48.5,FINESTEERING,2107,282733.950,02000000,471d,15824;INS_ALIGNMENT_COMPLETE,INS_RTKFIXED,37.37063924201,126.72426559710,10.4772,22.3000,0.2027,-0.2332,-0.0277,-0.317088293,-2.273099501,302.707061030,0.4435,0.2934,0.5506,0.1138,0.0925,0.0772,0.0985,0.1035,4.8550,0f000001,0*95b7724f\n\t", "INSPVAXA,USB3,0,48.5,FINESTEERING,2107,282734.450,02000000,471d,15824;INS_ALIGNMENT_COMPLETE,INS_RTKFIXED,37.37064005686,126.72426435901,10.4738,22.3000,0.1910,-0.2119,-0.0289,-0.216766474,-2.387675538,302.660035367,0.4432,0.2934,0.5508,0.1138,0.0925,0.0772,0.0985,0.1036,4.8555,0f000001,0*b9d42d58\n\t", "INSPVAXA,USB3,0,46.0,FINESTEERING,2107,282745.450,02000000,471d,15824;INS_ALIGNMENT_COMPLETE,INS_RTKFIXED,37.37065707294,126.72423583291,10.4038,22.3000,0.1644,-0.2205,-0.0248,-0.393666989,-2.802189375,301.368033402,0.4424,0.2935,0.5497,0.1137,0.0923,0.0771,0.0985,0.1035,4.8609,0f000001,0*4c364312\n\t", "INSPVAXA,USB3,0,50.5,FINESTEERING,2107,282766.000,02000000,471d,15824;INS_ALIGNMENT_COMPLETE,INS_RTKFIXED,37.37068918572,126.72418251405,10.1497,22.3000,0.1565,-0.2244,-0.0284,-1.470427926,-2.806836785,301.304662044,0.4416,0.2936,0.5519,0.1137,0.0923,0.0773,0.0984,0.1037,4.8731,0f000001,0*1edafe1a\n\t", "INSPVAXA,USB3,0,48.0,FINESTEERING,2107,282766.500,02000000,471d,15824;INS_ALIGNMENT_COMPLETE,INS_RTKFIXED,37.37068991155,126.72418127348,10.1440,22.3000,0.1660,-0.2361,-0.0346,-1.526557069,-2.043657004,301.319503447,0.4414,0.2936,0.5516,0.1147,0.0924,0.0773,0.0985,0.1037,4.8734,0f000001,0*5a4270f2\n\t", "INSPVAXA,USB3,0,52.5,FINESTEERING,2107,282769.500,02000000,471d,15824;INS_ALIGNMENT_COMPLETE,INS_RTKFIXED,37.37069431364,126.72417373673,10.1300,22.3000,0.1603,-0.2654,-0.0095,-1.268871738,-0.382060792,301.325978301,0.4464,0.2940,0.5510,0.1165,0.0927,0.0772,0.0984,0.1035,4.8643,0f000001,0*c8529f83\n\t", "INSPVAXA,USB3,0,50.5,FINESTEERING,2107,282771.500,02000000,471d,15824;INS_ALIGNMENT_COMPLETE,INS_RTKFIXED,37.37069745960,126.72416836041,10.1313,22.3000,0.1734,-0.2561,-0.0200,-1.398091128,-0.585991174,301.767912429,0.4476,0.2943,0.5503,0.1154,0.0929,0.0772,0.0983,0.1033,4.8370,0f000001,0*46dd6173\n\t", "INSPVAXA,USB3,0,48.0,FINESTEERING,2107,282774.000,02000000,471d,15824;INS_ALIGNMENT_COMPLETE,INS_RTKFIXED,37.37070158360,126.72416168804,10.1302,22.3000,0.1865,-0.2187,-0.0076,-0.878281232,-1.102464115,302.124757826,0.4458,0.2946,0.5497,0.1138,0.0924,0.0771,0.0982,0.1032,4.8072,0f000001,0*778beed4\n\t", "INSPVAXA,USB3,0,51.0,FINESTEERING,2107,282774.500,02000000,471d,15824;INS_ALIGNMENT_COMPLETE,INS_RTKFIXED,37.37070240562,126.72416038344,10.1301,22.3000,0.1841,-0.2216,-0.0074,-0.755916604,-1.039971548,302.079440422,0.4445,0.2942,0.5497,0.1137,0.0923,0.0771,0.0982,0.1032,4.7994,0f000001,0*7d8abcba\n\t", "INSPVAXA,USB3,0,52.0,FINESTEERING,2107,282777.000,02000000,471d,15824;INS_ALIGNMENT_COMPLETE,INS_RTKFIXED,37.37070657070,126.72415376285,10.1217,22.3000,0.2035,-0.2369,-0.0150,-0.446978250,-1.366804369,301.502448560,0.4425,0.2939,0.5496,0.1135,0.0924,0.0771,0.0982,0.1032,4.7938,0f000001,0*25f2a73f\n\t", "INSPVAXA,USB3,0,51.5,FINESTEERING,2107,282777.500,02000000,471d,15824;INS_ALIGNMENT_COMPLETE,INS_RTKFIXED,37.37070737696,126.72415245019,10.1203,22.3000,0.1993,-0.2523,-0.0201,-0.489054474,-1.485846051,301.354572444,0.4412,0.2937,0.5492,0.1134,0.0927,0.0771,0.0982,0.1032,4.7938,0f000001,0*c63e4195\n\t", "INSPVAXA,USB3,0,51.5,FINESTEERING,2107,282778.000,02000000,471d,15824;INS_ALIGNMENT_COMPLETE,INS_RTKFIXED,37.37070818895,126.72415111526,10.1183,22.3000,0.1970,-0.2381,-0.0048,-0.588842364,-1.719100289,301.162178179,0.4412,0.2937,0.5492,0.1134,0.0927,0.0771,0.0982,0.1032,4.7938,0f000001,0*cff0a9c3\n\t", "INSPVAXA,USB3,0,45.0,FINESTEERING,2107,282780.000,02000000,471d,15824;INS_ALIGNMENT_COMPLETE,INS_RTKFIXED,37.37071131338,126.72414591828,10.1018,22.3000,0.1785,-0.2324,-0.0069,-0.645891836,-1.424803808,300.174839081,0.4413,0.2936,0.5502,0.1138,0.0926,0.0771,0.0982,0.1032,4.7947,0f000001,0*1d8f369d\n\t", "INSPVAXA,USB3,0,47.0,FINESTEERING,2107,282780.500,02000000,471d,15824;INS_ALIGNMENT_COMPLETE,INS_RTKFIXED,37.37071208302,126.72414463488,10.0975,22.3000,0.1821,-0.2419,-0.0019,-0.556153794,-1.244614265,299.928543824,0.4419,0.2936,0.5508,0.1139,0.0925,0.0772,0.0982,0.1033,4.7946,0f000001,0*8f6fb982\n\t", "INSPVAXA,USB3,0,52.5,FINESTEERING,2107,282783.500,02000000,471d,15824;INS_ALIGNMENT_COMPLETE,INS_RTKFIXED,37.37071667102,126.72413686312,10.0669,22.3000,0.1872,-0.2243,-0.0265,-0.901347734,-1.882595886,299.189069382,0.4437,0.2938,0.5525,0.1145,0.0924,0.0772,0.0982,0.1033,4.7951,0f000001,0*f21a15f8\n\t", "INSPVAXA,USB3,0,52.5,FINESTEERING,2107,282784.000,02000000,471d,15824;INS_ALIGNMENT_COMPLETE,INS_RTKFIXED,37.37071744310,126.72413557177,10.0615,22.3000,0.1842,-0.2203,-0.0202,-0.879207865,-1.728416069,299.181717490,0.4437,0.2938,0.5525,0.1145,0.0924,0.0772,0.0982,0.1033,4.7951,0f000001,0*6c7250dc\n\t", "INSPVAXA,USB3,0,48.5,FINESTEERING,2107,282786.000,02000000,471d,15824;INS_ALIGNMENT_COMPLETE,INS_RTKFIXED,37.37072048781,126.72413033534,10.0312,22.3000,0.2068,-0.2374,-0.0322,-0.835692120,-1.272043539,298.989138355,0.4439,0.2941,0.5534,0.1141,0.0925,0.0773,0.0982,0.1033,4.7952,0f000001,0*6862fbb7\n\t", "INSPVAXA,USB3,0,50.0,FINESTEERING,2107,282786.500,02000000,471d,15824;INS_ALIGNMENT_COMPLETE,INS_RTKFIXED,37.37072125488,126.72412899591,10.0263,22.3000,0.1993,-0.2318,-0.0321,-0.677738340,-1.537504569,298.882185903,0.4440,0.2942,0.5536,0.1140,0.0923,0.0773,0.0982,0.1033,4.7960,0f000001,0*3cb3310e\n\t", "INSPVAXA,USB3,0,50.0,FINESTEERING,2107,282787.000,02000000,471d,15824;INS_ALIGNMENT_COMPLETE,INS_RTKFIXED,37.37072202374,126.72412763229,10.0205,22.3000,0.2013,-0.2217,-0.0210,-0.794961813,-1.788062217,298.885711292,0.4440,0.2942,0.5536,0.1140,0.0923,0.0773,0.0982,0.1033,4.7960,0f000001,0*1f81862e\n\t", "INSPVAXA,USB3,0,44.0,FINESTEERING,2107,282787.500,02000000,471d,15824;INS_ALIGNMENT_COMPLETE,INS_RTKFIXED,37.37072277220,126.72412626224,10.0147,22.3000,0.2002,-0.2137,-0.0290,-0.849980745,-1.812919554,298.887708696,0.4445,0.2943,0.5539,0.1141,0.0924,0.0773,0.0982,0.1034,4.7971,0f000001,0*c9e15001\n\t", "INSPVAXA,USB3,0,44.0,FINESTEERING,2107,282788.000,02000000,471d,15824;INS_ALIGNMENT_COMPLETE,INS_RTKFIXED,37.37072352565,126.72412491087,10.0076,22.3000,0.2060,-0.2242,-0.0325,-0.865126530,-1.802719391,298.872730955,0.4445,0.2943,0.5539,0.1141,0.0924,0.0773,0.0982,0.1034,4.7971,0f000001,0*c2266642\n\t", "INSPVAXA,USB3,0,49.0,FINESTEERING,2107,282788.500,02000000,471d,15824;INS_ALIGNMENT_COMPLETE,INS_RTKFIXED,37.37072428040,126.72412354813,10.0007,22.3000,0.2098,-0.2286,-0.0305,-0.732817876,-1.872220332,298.881417220,0.4449,0.2943,0.5542,0.1142,0.0924,0.0773,0.0982,0.1034,4.7982,0f000001,0*a1e1a8aa\n\t", "INSPVAXA,USB3,0,49.0,FINESTEERING,2107,282789.000,02000000,471d,15824;INS_ALIGNMENT_COMPLETE,INS_RTKFIXED,37.37072504347,126.72412218219,9.9929,22.3000,0.1951,-0.2277,-0.0250,-0.679984989,-2.019858796,298.956218881,0.4449,0.2943,0.5542,0.1142,0.0924,0.0773,0.0982,0.1034,4.7982,0f000001,0*d14e3525\n\t", "INSPVAXA,USB3,0,50.5,FINESTEERING,2107,282789.500,02000000,471d,15824;INS_ALIGNMENT_COMPLETE,INS_RTKFIXED,37.37072577695,126.72412082127,9.9869,22.3000,0.2017,-0.2348,-0.0299,-0.707518535,-2.196709608,298.969096628,0.4457,0.2945,0.5546,0.1143,0.0924,0.0773,0.0982,0.1035,4.7994,0f000001,0*e2b500de\n\t", "INSPVAXA,USB3,0,50.5,FINESTEERING,2107,282790.000,02000000,471d,15824;INS_ALIGNMENT_COMPLETE,INS_RTKFIXED,37.37072651838,126.72411947234,9.9801,22.3000,0.2152,-0.2350,-0.0246,-0.689288795,-2.210478200,298.973213622,0.4457,0.2945,0.5546,0.1143,0.0924,0.0773,0.0982,0.1035,4.7994,0f000001,0*67dd8a4d\n\t", "INSPVAXA,USB3,0,50.0,FINESTEERING,2107,282790.500,02000000,471d,15824;INS_ALIGNMENT_COMPLETE,INS_RTKFIXED,37.37072725997,126.72411813576,9.9737,22.3000,0.1949,-0.2238,-0.0215,-0.636862822,-2.266623064,299.084984877,0.4461,0.2946,0.5548,0.1144,0.0925,0.0773,0.0983,0.1035,4.8006,0f000001,0*d9aa8359\n\t", "DUALANTENNAHEADINGA,USB3,0,50.0,FINESTEERING,2107,282791.000,02000000,d426,15824;INSUFFICIENT_OBS,NONE,-1.000000000,0.000000000,0.000000000,0.0,0.000000000,0.000000000,\"631T\",14,2,2,2,04,00,20,00*cf3d8ad9\n\t", "INSPVAXA,USB3,0,49.0,FINESTEERING,2107,282791.500,02000000,471d,15824;INS_ALIGNMENT_COMPLETE,INS_RTKFIXED,37.37072877959,126.72411543719,9.9612,22.3000,0.2083,-0.2487,-0.0306,-0.425657916,-2.232797757,299.196171617,0.4458,0.2943,0.5547,0.1143,0.0925,0.0773,0.0983,0.1035,4.8018,0f000001,0*f23e3c59\n\t", "INSPVAXA,USB3,0,49.0,FINESTEERING,2107,282792.000,02000000,471d,15824;INS_ALIGNMENT_COMPLETE,INS_RTKFIXED,37.37072953138,126.72411411925,9.9544,22.3000,0.1984,-0.2313,-0.0308,-0.400223692,-2.232054336,299.272403656,
